vi "HWSync Cmd Dialog.vi"(8 "error in (no error)":errorcluster, 10 "Log Queue":refnum<queue>, 11 "Hal Queue in":refnum<queue>) -> (0 "error out":errorcluster, 2 "Msg out":string)   [LabVIEW 2014]
uses:
  APIs/Message Queue/Message Cluster.ctl
  APIs/Message Queue/Enqueue Message (Single).vi
  APIs/Message Queue/Enqueue Message (Array).vi
  APIs/Message Queue/WINFAS 2 Message Queue.lvlib
panel:
  in  "Encoder Zero":bool
  in  "DO":bool[][](array[boolean])=[[FALSE, FALSE, FALSE, FALSE, FALSE, FALSE, FALSE, FALSE], [FALSE, FALSE, FALSE, FALSE, FALSE, FALSE, FALSE, FALSE]]
  in  "Measurement Stop":bool
  in  "Write Outputs":bool
  in  "Measurement Start":bool
  in  "HWSincrono 5":bool
  in  "HWSincrono 4":bool
  in  "HWSincrono 3":bool
  in  "HWSincrono 2":bool
  in  "HWSincrono 1":bool
  # "Hardware Síncrono #"
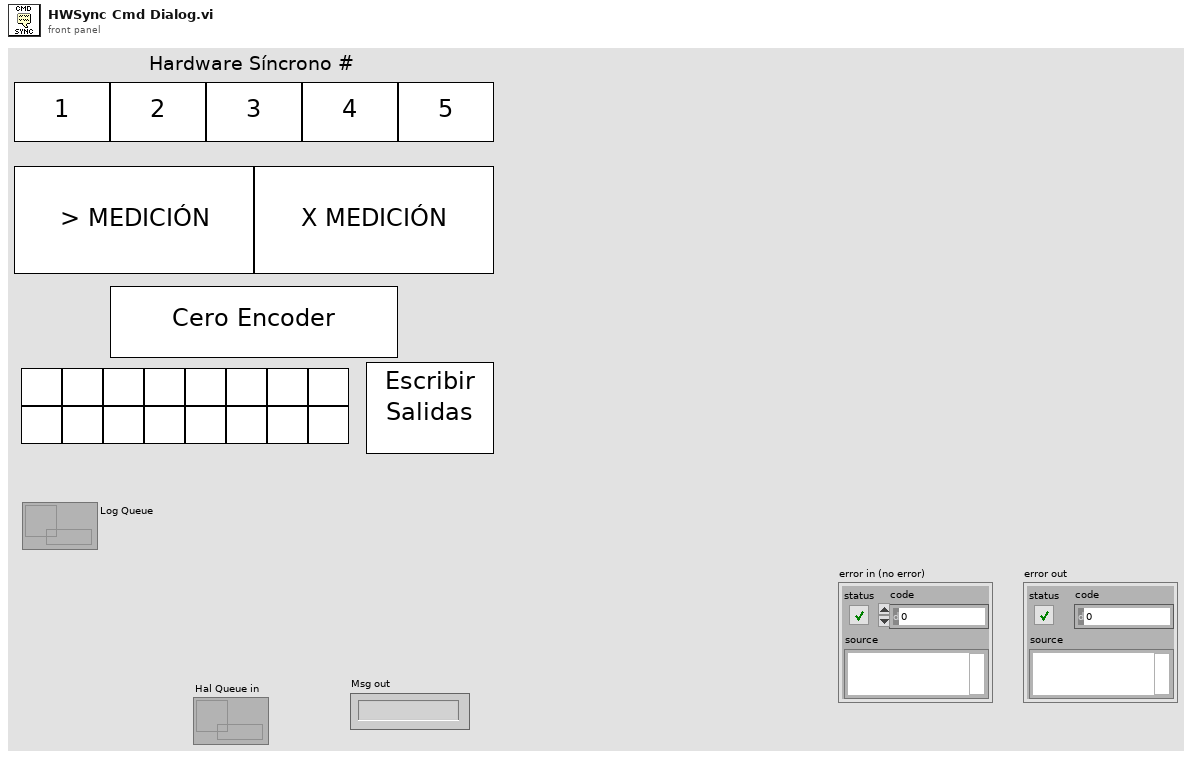
[diagram p1: front panel]
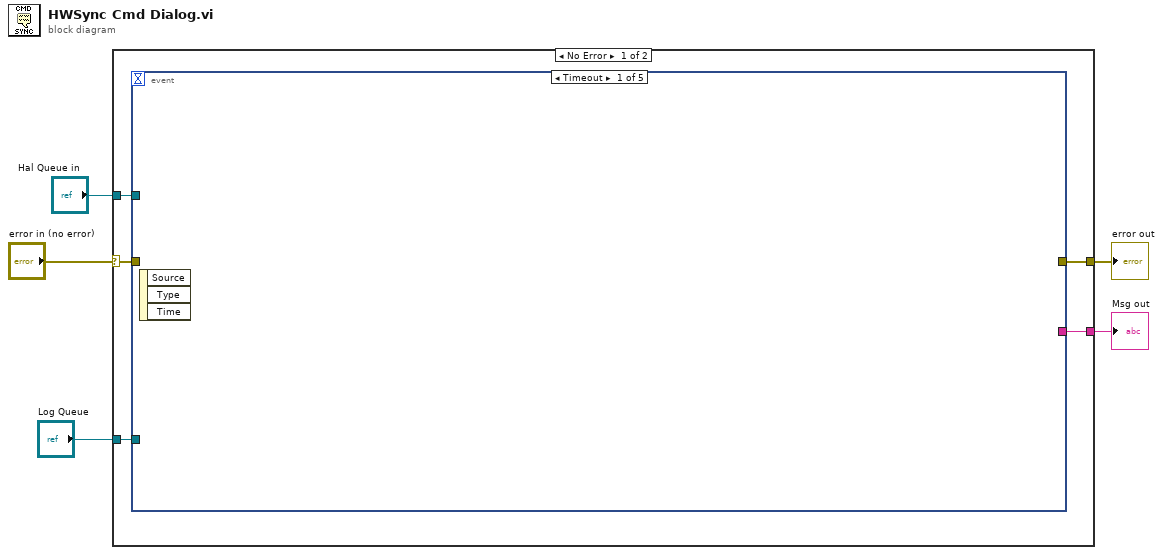
[diagram p0: block diagram]
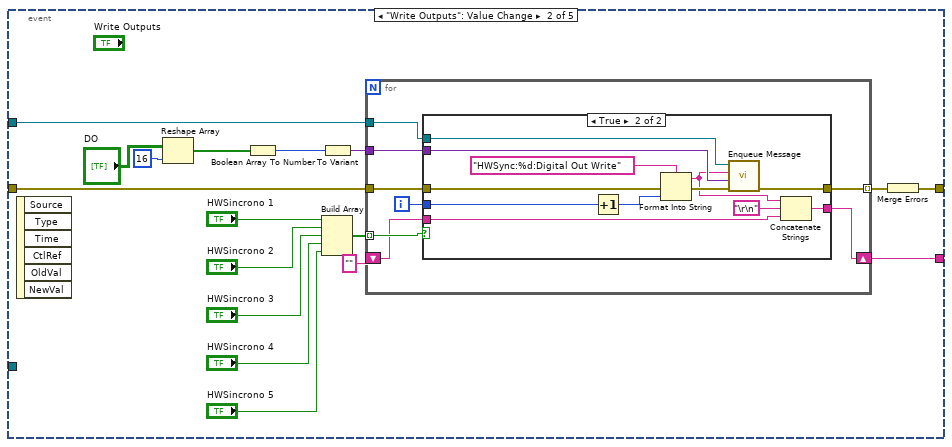
[diagram p2: hidden frame]
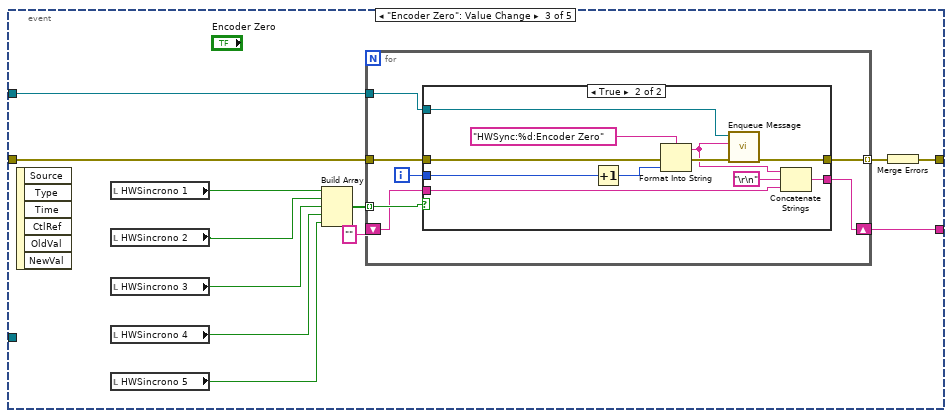
[diagram p4: hidden frame]
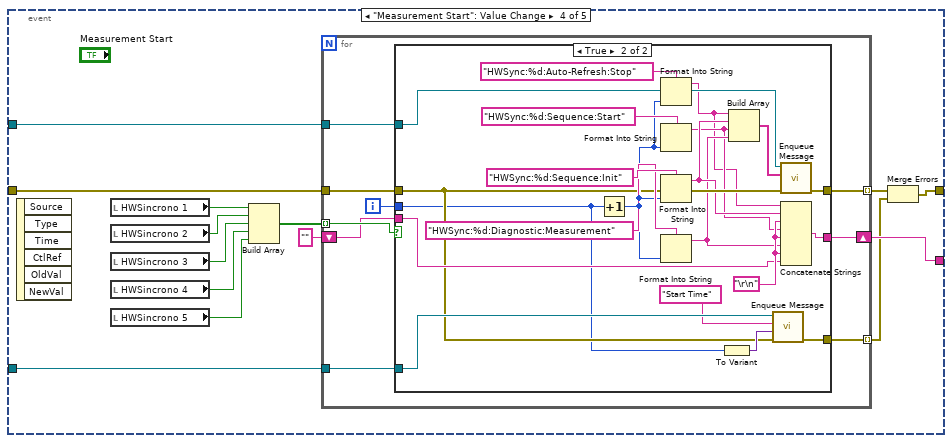
[diagram p6: hidden frame]
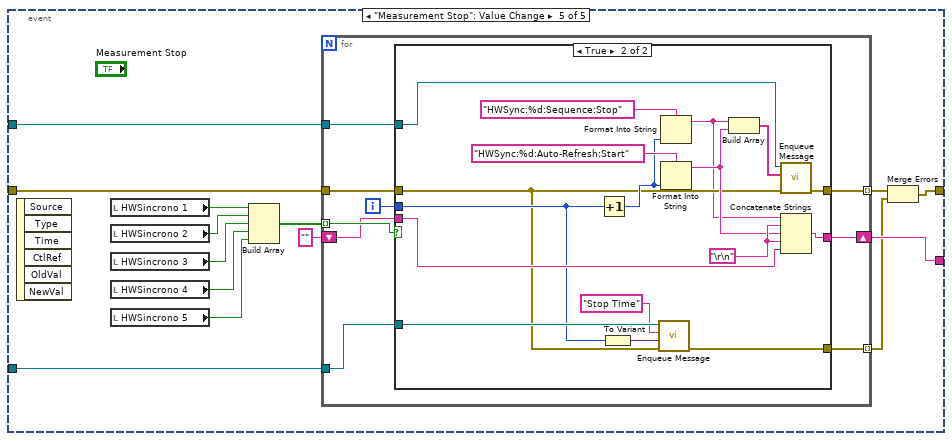
[diagram p8: hidden frame]
diagram:
  n1 = case shown="No Error" "error in (no error)" {
    selector: "error in (no error)" -> [w9 w171]
    tunnel: [w8 w171] -> w5
    tunnel: "Hal Queue in" -> [w10 _]
    tunnel: [w7 _] -> w2
    tunnel: "Log Queue" -> [w6 _]
    frame No Error {
      n2 = event shown="[0] Timeout" {
        selector: _ -> [_ _ _ _ _]
        dyn-events: _ -> [_ _ _ _ _]
        timeout: _ -> [_ _ _ _ _]
        tunnel: w10 -> [_ w14 w58 w92 w139]
        tunnel: w9 -> [_ w18 w61 w95 w142]
        tunnel: [_ w15 w59 w93 w140] -> w8
        tunnel: [_ w12 w56 w85 w132] -> w7
        tunnel: w6 -> [_ _ _ w83 w130]
        event Timeout {
          n3 = event-data() -> ()  [unwired: 1 in, 3 out]
        }
        event "Write Outputs": Value Change {
          n4 = event-data() -> ()  [unwired: 1 in, 6 out]
          n5 = Reshape Array("DO", 16 ("dimension size")) -> (w25:bool[])
          n6 = Boolean Array To Number(Boolean array=w25) -> (number=w24:u32)
          n7 = Build Array("HWSincrono 1", "HWSincrono 2", "HWSincrono 3", "HWSincrono 4", "HWSincrono 5") -> (w13:bool[])
          n8 = To Variant(anything=w24) -> (Variant=w17:variant)
          n9 = for {
            tunnel: w18 -> [w32]
            tunnel: w17 -> [w35]
            tunnel: [w34] -> w16 mode=indexing
            tunnel: w14 -> [w33]
            tunnel: w13 -> [w30] mode=indexing
            shift-right: [w29] -> w12
            shift-left: "" -> [w28]
            i -> [w31]
            n10 = case shown="True" w30 {
              tunnel: w35 -> [_ w49]
              tunnel: [w37 w47] -> w34
              tunnel: w33 -> [_ w46]
              tunnel: w32 -> [w37 w44]
              tunnel: w31 -> [_ w43]
              tunnel: [w36 w39] -> w29
              tunnel: w28 -> [w36 w38]
              frame False {
              }
              frame True {
                n11 = Increment(x=w43) -> (x+1=w42:i32)
                n12 = Format Into String(format string="HWSync:%d:Digital Out Write", error in=w44, w42) -> (resulting string=w41:string, error out=w45:errorcluster)  [unwired: 1 in]
                n13 = call-poly "Enqueue Message.vi"("error in (no error)"=w45, "Message Data"=w49, "Message"=w41, "Message Queue"=w46) -> ("error out"=w47:errorcluster)  [unwired: 6 in, 1 out]
                n14 = Concatenate Strings(w41, "\r\n", w38) -> (w39:string)
              }
            }
          }
          n15 = Merge Errors(w16) -> (w15:errorcluster)
        }
        event "Encoder Zero": Value Change {
          n16 = event-data() -> ()  [unwired: 1 in, 6 out]
          n17 = local read "HWSincrono 1"() -> (w54:bool)
          n18 = local read "HWSincrono 2"() -> (w53:bool)
          n19 = local read "HWSincrono 3"() -> (w52:bool)
          n20 = local read "HWSincrono 4"() -> (w51:bool)
          n21 = local read "HWSincrono 5"() -> (w50:bool)
          n22 = Build Array(w54, w53, w52, w51, w50) -> (w57:bool[])
          n23 = for {
            tunnel: w61 -> [w66]
            tunnel: [w68] -> w60 mode=indexing
            tunnel: w58 -> [w67]
            tunnel: w57 -> [w64] mode=indexing
            shift-right: [w63] -> w56
            shift-left: "" -> [w62]
            i -> [w65]
            n24 = case shown="True" w64 {
              tunnel: [w70 w80] -> w68
              tunnel: w67 -> [_ w79]
              tunnel: w66 -> [w70 w77]
              tunnel: w65 -> [_ w76]
              tunnel: [w69 w72] -> w63
              tunnel: w62 -> [w69 w71]
              frame False {
              }
              frame True {
                n25 = Increment(x=w76) -> (x+1=w75:i32)
                n26 = Format Into String(format string="HWSync:%d:Encoder Zero", error in=w77, w75) -> (resulting string=w74:string, error out=w78:errorcluster)  [unwired: 1 in]
                n27 = call-poly "Enqueue Message.vi"("error in (no error)"=w78, "Message"=w74, "Message Queue"=w79) -> ("error out"=w80:errorcluster)  [unwired: 7 in, 1 out]
                n28 = Concatenate Strings(w74, "\r\n", w71) -> (w72:string)
              }
            }
          }
          n29 = Merge Errors(w60) -> (w59:errorcluster)
        }
        event "Measurement Start": Value Change {
          n30 = event-data() -> ()  [unwired: 1 in, 6 out]
          n31 = local read "HWSincrono 1"() -> (w90:bool)
          n32 = local read "HWSincrono 2"() -> (w89:bool)
          n33 = local read "HWSincrono 3"() -> (w88:bool)
          n34 = local read "HWSincrono 4"() -> (w87:bool)
          n35 = local read "HWSincrono 5"() -> (w86:bool)
          n36 = Build Array(w90, w89, w88, w87, w86) -> (w91:bool[])
          n37 = for {
            tunnel: w95 -> [w102]
            tunnel: [w104] -> w94 mode=indexing
            tunnel: w92 -> [w103]
            tunnel: w91 -> [w100] mode=indexing
            shift-right: [w99] -> w85
            shift-left: "" -> [w98]
            tunnel: w83 -> [w97]
            tunnel: [w96] -> w82 mode=indexing
            i -> [w101]
            n38 = case shown="True" w100 {
              tunnel: [w105 w127] -> w104
              tunnel: w103 -> [_ w126]
              tunnel: w102 -> [w105 w109]
              tunnel: w101 -> [_ w108]
              tunnel: [w106 w118] -> w99
              tunnel: w98 -> [w106 w117]
              tunnel: w97 -> [_ w113]
              tunnel: [w105 w110] -> w96
              frame False {
              }
              frame True {
                w120 = "\r\n"
                n39 = Increment(x=w108) -> (x+1=w114:i32)
                n40 = Format Into String(format string="HWSync:%d:Auto-Refresh:Stop", w114) -> (resulting string=w107:string)  [unwired: 2 in, 1 out]
                n41 = Format Into String(format string="HWSync:%d:Sequence:Start", w114) -> (resulting string=w115:string)  [unwired: 2 in, 1 out]
                n42 = Format Into String(format string="HWSync:%d:Sequence:Init", error in=w109, w114) -> (resulting string=w121:string, error out=w125:errorcluster)  [unwired: 1 in]
                n43 = Format Into String(format string="HWSync:%d:Diagnostic:Measurement", w114) -> (resulting string=w119:string)  [unwired: 2 in, 1 out]
                n44 = To Variant(anything=w108) -> (Variant=w111:variant)
                n45 = Build Array(w107, w121, w115, w119) -> (w124:string[])
                n46 = call-poly "Enqueue Message.vi"("error in (no error)"=w109, "Message Data"=w111, "Message"="Start Time", "Message Queue"=w113) -> ("error out"=w110:errorcluster)  [unwired: 6 in, 1 out]
                n47 = call-poly "Enqueue Message.vi"("error in (no error)"=w125, "Message Array"=w124, "Message Queue"=w126) -> ("error out"=w127:errorcluster)  [unwired: 7 in, 1 out]
                n48 = Concatenate Strings(w107, w121, w120, w115, w120, w119, w120, w117) -> (w118:string)
              }
            }
          }
          n49 = Merge Errors(w94, w82) -> (w93:errorcluster)
        }
        event "Measurement Stop": Value Change {
          n50 = event-data() -> ()  [unwired: 1 in, 6 out]
          n51 = local read "HWSincrono 1"() -> (w137:bool)
          n52 = local read "HWSincrono 2"() -> (w136:bool)
          n53 = local read "HWSincrono 3"() -> (w135:bool)
          n54 = local read "HWSincrono 4"() -> (w134:bool)
          n55 = local read "HWSincrono 5"() -> (w133:bool)
          n56 = Build Array(w137, w136, w135, w134, w133) -> (w138:bool[])
          n57 = for {
            tunnel: w142 -> [w149]
            tunnel: [w151] -> w141 mode=indexing
            tunnel: w139 -> [w150]
            tunnel: w138 -> [w147] mode=indexing
            shift-right: [w146] -> w132
            shift-left: "" -> [w145]
            tunnel: w130 -> [w144]
            tunnel: [w143] -> w129 mode=indexing
            i -> [w148]
            n58 = case shown="True" w147 {
              tunnel: [w152 w170] -> w151
              tunnel: w150 -> [_ w169]
              tunnel: w149 -> [w152 w157]
              tunnel: w148 -> [_ w158]
              tunnel: [w153 w165] -> w146
              tunnel: w145 -> [w153 w161]
              tunnel: w144 -> [_ w159]
              tunnel: [w152 w154] -> w143
              frame False {
              }
              frame True {
                w166 = "\r\n"
                n59 = Increment(x=w158) -> (x+1=w162:i32)
                n60 = To Variant(anything=w158) -> (Variant=w160:variant)
                n61 = call-poly "Enqueue Message.vi"("error in (no error)"=w157, "Message Data"=w160, "Message"="Stop Time", "Message Queue"=w159) -> ("error out"=w154:errorcluster)  [unwired: 6 in, 1 out]
                n62 = Format Into String(format string="HWSync:%d:Sequence:Stop", w162) -> (resulting string=w156:string)  [unwired: 2 in, 1 out]
                n63 = Format Into String(format string="HWSync:%d:Auto-Refresh:Start", w162) -> (resulting string=w163:string)  [unwired: 2 in, 1 out]
                n64 = Build Array(w156, w163) -> (w168:string[])
                n65 = call-poly "Enqueue Message.vi"("error in (no error)"=w157, "Message Array"=w168, "Message Queue"=w169) -> ("error out"=w170:errorcluster)  [unwired: 7 in, 1 out]
                n66 = Concatenate Strings(w156, w166, w163, w166, w161) -> (w165:string)
              }
            }
          }
          n67 = Merge Errors(w141, w129) -> (w140:errorcluster)
        }
      }
    }
    frame Error {
    }
  }
  "error out" <- w5
  "Msg out" <- w2
